vi "LV10_4a.vi"() -> ()   [LabVIEW 2014]
uses:
  <vilib>/picture/picture.llb/Draw 8-Bit Pixmap.vi
panel:
  in  "Stages":u16(ring) items=["1", "2", "3", "4"]
  out "Haar wavelet transform":picture
  out "Original image":picture
  in  "Stop Button":bool
  out "Reconstructed image":picture
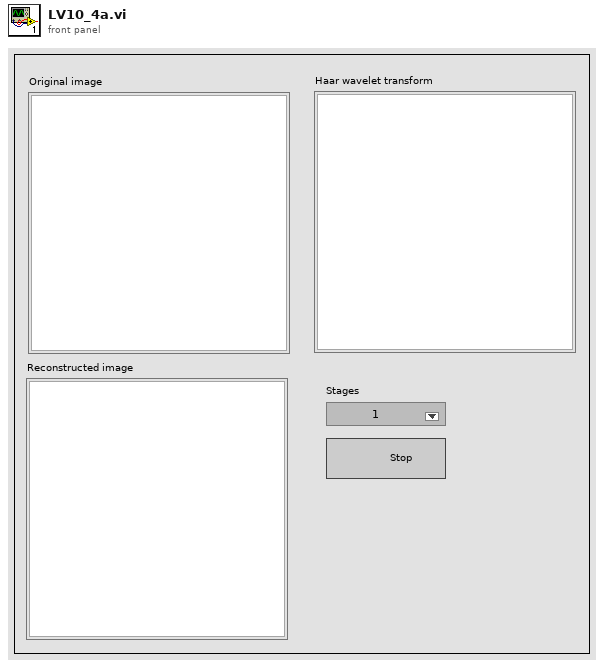
[diagram p1: front panel]
types:
  T1 = typedef "imagedata.ctl" = cluster{"image type":i32, "image depth":i32, "image":u8[], "mask":u8[], "colors":u32[], "Rectangle":cluster{"left":i16, "top":i16, "right":i16, "bottom":i16}}
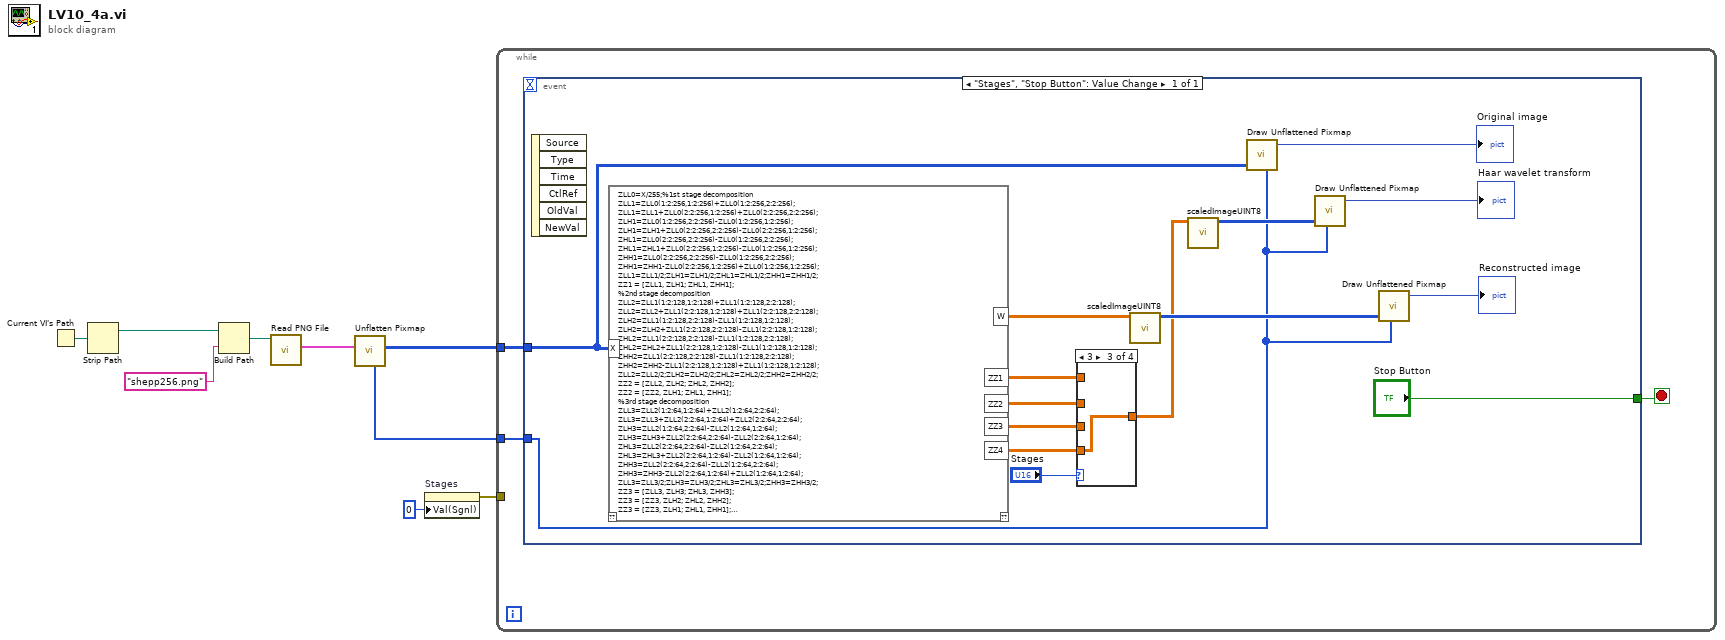
[diagram p0: block diagram]
diagram:
  n1 = Current VI's Path() -> (path=w9:path)
  n2 = Strip Path(path=w9) -> (stripped path=w1:path)  [unwired: 1 out]
  n3 = Build Path(base path=w1, name or relative path="shepp256.png") -> (appended path=w6:path)
  n4 = call <vilib>:"Read PNG File.vi"("path to PNG file"=w6) -> ("image data"=w5:T1)  [unwired: 8 in, 2 out]
  n5 = call <vilib>:"Unflatten Pixmap.vi"("image data"=w5) -> ("8-bit pixmap"=w7:u8[][], "colors"=w4:u32[])  [unwired: 4 in, 5 out]
  n6 = property on="Stages" class="Ring (strict)"("Val(Sgnl)"=u16 0 ("Value (Signaling)")) -> (error out=w3:errorcluster)  [unwired: 2 in, 1 out]
  n7 = while {
    tunnel: w7 -> [w11]
    tunnel: w4 -> [w10]
    tunnel: w3 -> [_]
    stop <- w12 stop-if-true
    n8 = event shown="[0] \"Stages\", \"Stop Button\": Value Change" {
      selector: _ -> [_]
      dyn-events: _ -> [_]
      timeout: _ -> [_]
      tunnel: ["Stop Button"] -> w12
      tunnel: w11 -> [w24]
      tunnel: w10 -> [w19]
      event "Stages", "Stop Button": Value Change {
        n9 = event-data() -> ()  [unwired: 1 in, 6 out]
        n10 = mathscript code="ZLL0=X/255;%1st stage decomposition\nZLL1=ZLL0(1:2:256,1:2:256)+ZLL0(1:2:256,2:2:256);\nZLL1=ZLL1+ZLL0(2:2:256,1:2:256)+ZLL0(2:2:256,2:2:256);\nZLH1=ZLL0(1:2:256,2:2:256)-ZLL0(1:2:256,1:2:256);\nZLH1=ZLH1+ZLL0(2:2:256,2:2:256)-ZLL0(2:2:256,1:2:256);\nZHL1=ZLL0(2:2:256,2:2:256)-ZLL0(1:2:256,2:2:256);\nZHL1=ZHL1+ZLL0(2:2:256,1:2:256)-ZLL0(1:2:256,1:2:256);\nZHH1=ZLL0(2:2:256,2:2:256)-ZLL0(1:2:256,2:2:256);\nZHH1=ZHH1-ZLL0(2:2:256,1:2:256)+ZLL0(1:2:256,1:2:256);\nZLL1=ZLL1/2;ZLH1=ZLH1/2;ZHL1=ZHL1/2;ZHH1=ZHH1/2;\nZZ1 = [ZLL1, ZLH1; ZHL1, ZHH1];\n%2nd stage decomposition\nZLL2=ZLL1(1:2:128,1:2:128)+ZLL1(1:2:128,2:2:128);\nZLL2=ZLL2+ZLL1(2:2:128,1:2:128)+ZLL1(2:2:128,2:2:128);\nZLH2=ZLL1(1:2:128,2:2:128)-ZLL1(1:2:128,1:2:128);\nZLH2=ZLH2+ZLL1(2:2:128,2:2:128)-ZLL1(2:2:128,1:2:128);\nZHL2=ZLL1(2:2:128,2:2:128)-ZLL1(1:2:128,2:2:128);\nZHL2=ZHL2+ZLL1(2:2:128,1:2:128)-ZLL1(1:2:128,1:2:128);\nZHH2=ZLL1(2:2:128,2:2:128)-ZLL1(1:2:128,2:2:128);\nZHH2=ZHH2-ZLL1(2:2:128,1:2:128)+ZLL1(1:2:128,1:2:128);\nZLL2=ZLL2/2;ZLH2=ZLH2/2;ZHL2=ZHL2/2;ZHH2=ZHH2/2;\nZZ2 = [ZLL2, ZLH2; ZHL2, ZHH2];\nZZ2 = [ZZ2, ZLH1; ZHL1, ZHH1];\n%3rd stage decomposition\nZLL3=ZLL2(1:2:64,1:2:64)+ZLL2(1:2:64,2:2:64);\nZLL3=ZLL3+ZLL2(2:2:64,1:2:64)+ZLL2(2:2:64,2:2:64);\nZLH3=ZLL2(1:2:64,2:2:64)-ZLL2(1:2:64,1:2:64);\nZLH3=ZLH3+ZLL2(2:2:64,2:2:64)-ZLL2(2:2:64,1:2:64);\nZHL3=ZLL2(2:2:64,2:2:64)-ZLL2(1:2:64,2:2:64);\nZHL3=ZHL3+ZLL2(2:2:64,1:2:64)-ZLL2(1:2:64,1:2:64);\nZHH3=ZLL2(2:2:64,2:2:64)-ZLL2(1:2:64,2:2:64);\nZHH3=ZHH3-ZLL2(2:2:64,1:2:64)+ZLL2(1:2:64,1:2:64);\nZLL3=ZLL3/2;ZLH3=ZLH3/2;ZHL3=ZHL3/2;ZHH3=ZHH3/2;\nZZ3 = [ZLL3, ZLH3; ZHL3, ZHH3];\nZZ3 = [ZZ3, ZLH2; ZHL2, ZHH2];\nZZ3 = [ZZ3, ZLH1; ZHL1, ZHH1];\n%4th stage decomposition\nZLL4=ZLL3(1:2:32,1:2:32)+ZLL3(1:2:32,2:2:32);\nZLL4=ZLL4+ZLL3(2:2:32,1:2:32)+ZLL3(2:2:32,2:2:32);\nZLH4=ZLL3(1:2:32,2:2:32)-ZLL3(1:2:32,1:2:32);\nZLH4=ZLH4+ZLL3(2:2:32,2:2:32)-ZLL3(2:2:32,1:2:32);\nZHL4=ZLL3(2:2:32,2:2:32)-ZLL3(1:2:32,2:2:32);\nZHL4=ZHL4+ZLL3(2:2:32,1:2:32)-ZLL3(1:2:32,1:2:32);\nZHH4=ZLL3(2:2:32,2:2:32)-ZLL3(1:2:32,2:2:32);\nZHH4=ZHH4-ZLL3(2:2:32,1:2:32)+ZLL3(1:2:32,1:2:32);\nZLL4=ZLL4/2;ZLH4=ZLH4/2;ZHL4=ZHL4/2;ZHH4=ZHH4/2;\nZZ4=[ZLL4 ZLH4;ZHL4 ZHH4];%Display as image:\nZZ4=[ZZ4 ZLH3;ZHL3 ZHH3];\nZZ4=[ZZ4 ZLH2;ZHL2 ZHH2];\nZZ4=[ZZ4 ZLH1;ZHL1 ZHH1];\n\n%Inverse Haar (note double reversals, & FAST):\nWLL2(2:2:64,2:2:64)=(ZLL3+ZLH3+ZHL3+ZHH3)/2;\nWLL2(2:2:64,1:2:64)=(ZLL3-ZLH3+ZHL3-ZHH3)/2;\nWLL2(1:2:64,2:2:64)=(ZLL3+ZLH3-ZHL3-ZHH3)/2;\nWLL2(1:2:64,1:2:64)=(ZLL3-ZLH3-ZHL3+ZHH3)/2;\n%2nd stage:\nWLL1(2:2:128,2:2:128)=(WLL2+ZLH2+ZHL2+ZHH2)/2;\nWLL1(2:2:128,1:2:128)=(WLL2-ZLH2+ZHL2-ZHH2)/2;\nWLL1(1:2:128,2:2:128)=(WLL2+ZLH2-ZHL2-ZHH2)/2;\nWLL1(1:2:128,1:2:128)=(WLL2-ZLH2-ZHL2+ZHH2)/2;\n%1st stage:\nW(2:2:256,2:2:256)=(WLL1+ZLH1+ZHL1+ZHH1)/2;\nW(2:2:256,1:2:256)=(WLL1-ZLH1+ZHL1-ZHH1)/2;\nW(1:2:256,2:2:256)=(WLL1+ZLH1-ZHL1-ZHH1)/2;\nW(1:2:256,1:2:256)=(WLL1-ZLH1-ZHL1+ZHH1)/2;"("X"=w24) -> ("W"=w21:dbl[][], "ZZ4"=w15:dbl[][], "ZZ1"=w17:dbl[][], "ZZ2"=w16:dbl[][], "ZZ3"=w13:dbl[][])  [unwired: 1 in, 1 out]
        n11 = case shown="3" "Stages" {
          tunnel: w17 -> [_ _ _ w31]
          tunnel: w16 -> [w28 _ _ _]
          tunnel: w15 -> [_ _ w30 _]
          tunnel: [w28 w29 w30 w31] -> w14
          tunnel: w13 -> [_ w29 _ _]
          frame 1 {
          }
          frame 2 {
          }
          frame 3 {
          }
          frame 0, Default {
          }
        }
        n12 = call "scaledImageUINT8.vi"("double image"=w21) -> ("uint8 image"=w20:u8[][])  [unwired: 10 in]
        n13 = call "scaledImageUINT8.vi"("double image"=w14) -> ("uint8 image"=w22:u8[][])  [unwired: 10 in]
        n14 = call-poly <vilib>:"Draw Unflattened Pixmap.vi"("data"=w24, "color table"=w19) -> ("new picture"=→"Original image":picture)  [unwired: 7 in]
        n15 = call-poly <vilib>:"Draw Unflattened Pixmap.vi"("data"=w22, "color table"=w19) -> ("new picture"=→"Haar wavelet transform":picture)  [unwired: 7 in]
        n16 = call-poly <vilib>:"Draw Unflattened Pixmap.vi"("data"=w20, "color table"=w19) -> ("new picture"=→"Reconstructed image":picture)  [unwired: 7 in]
      }
    }
  }
